vi "PneumaticControl.vi"(1 "Device/Ports/Lines":string="Dev1/port2/line2\n", 2 "On/Off":bool, 3 "error in":errorcluster) -> (10 "error out":errorcluster)   [LabVIEW 2015]
panel:
  # "True means close relay"
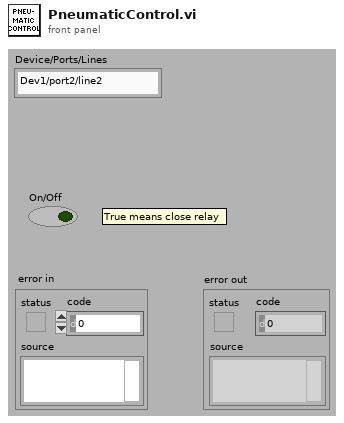
[diagram p1: front panel]
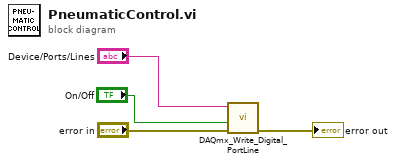
[diagram p0: block diagram]
diagram:
  n1 = call "DAQmx_Write_Digital_PortLine.vi"("Device/Ports/Lines"="Device/Ports/Lines", "Boolean"="On/Off", "error in"="error in") -> ("error out"=→"error out":errorcluster)  [unwired: 6 in, 1 out]
